vi "semafory.vi"() -> ()   [LabVIEW 2014]
uses:
  semafor.ctl
  #status.ctl
  semafor_tab.ctl
panel:
  in  "stop":bool
  in  "Do":i32
  in  "Od":i32
  out "Semafor S":T1
  out "Semafor  E":T1
  out "Semafor W":T1
  out "Semafor N":T1
  # "Noc"
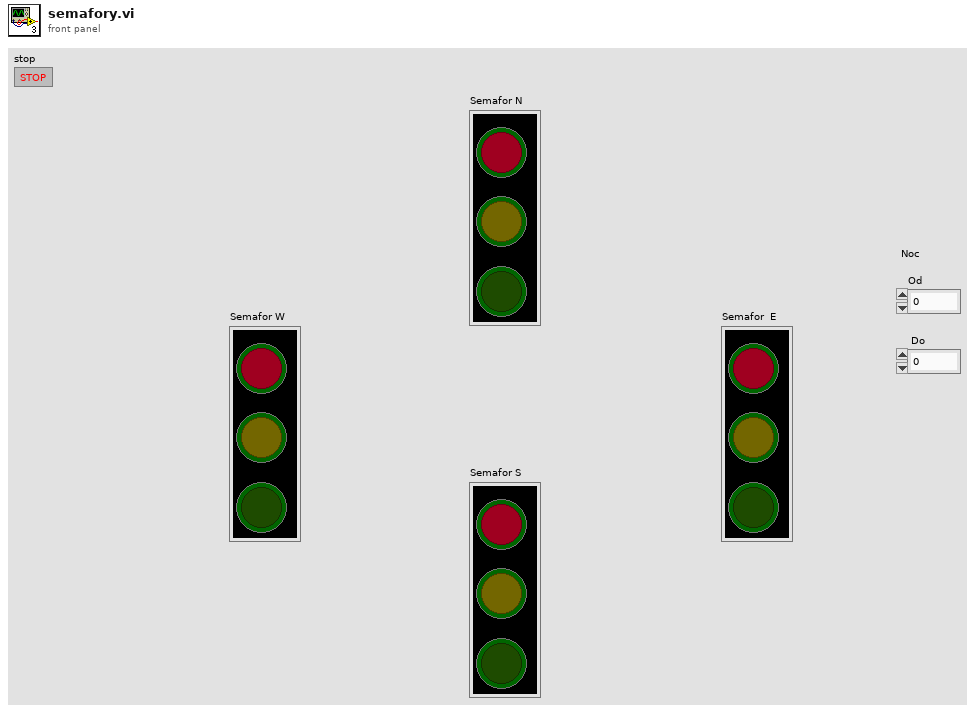
[diagram p1: front panel]
types:
  T1 = typedef "semafor.ctl" = cluster{"Y":bool, "G":bool, "R":bool}
  T2 = typedef "#status.ctl" = enum16{"Error_under_range", "Init", "Idle", "Night", "E-W-R", "E-W-Y", "E-W-G", "N-S-R", "N-S-Y", "N-S-G", "Exit"}
  T3 = typedef "semafor_tab.ctl" = cluster{"N":T1, "S":T1, "W":T1, "E":T1, "Time R ":dbl, "Time  Y":dbl, "Time  G":dbl}
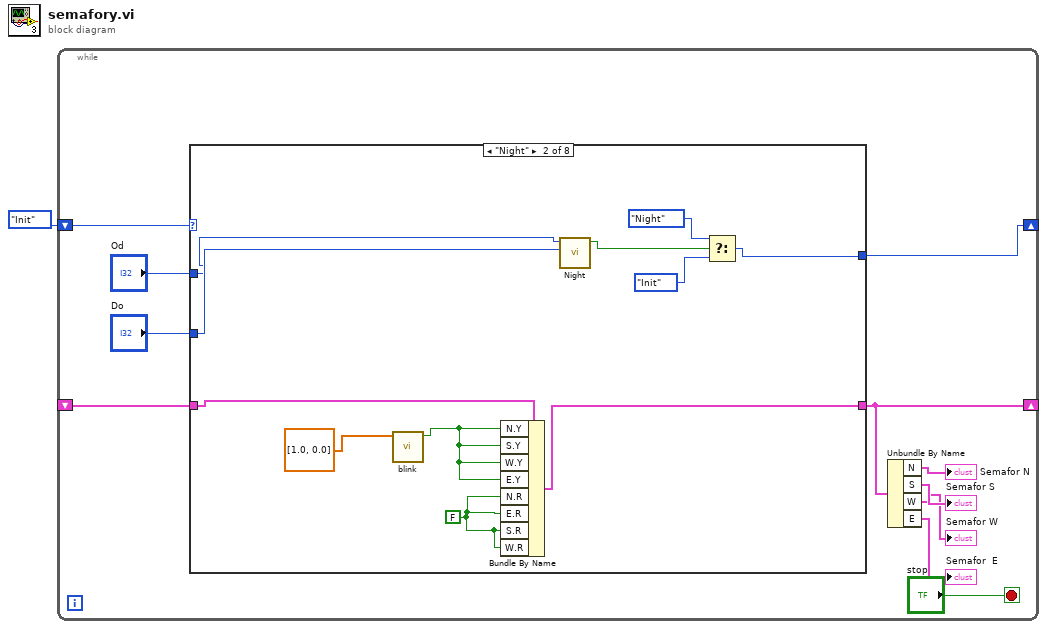
[diagram p0: block diagram]
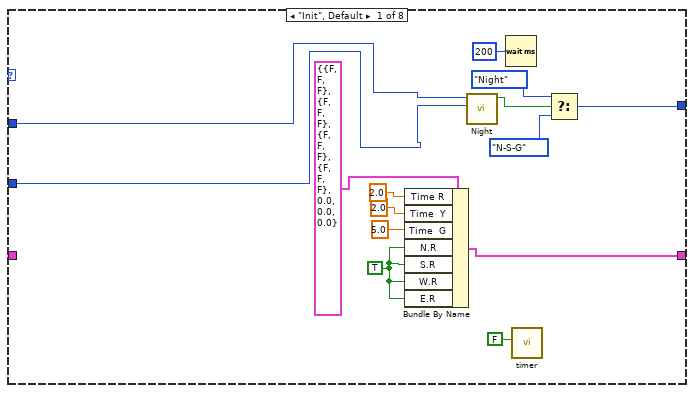
[diagram p2: hidden frame]
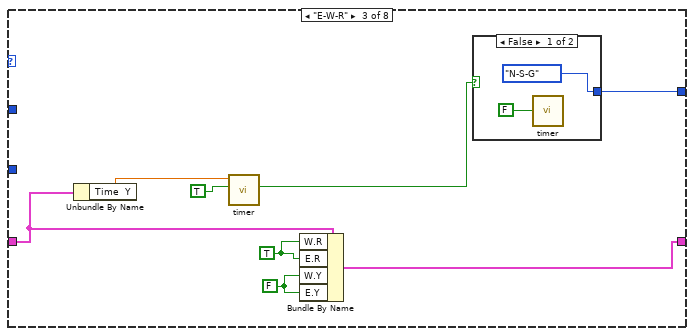
[diagram p3: hidden frame]
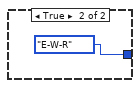
[diagram p4: hidden frame]
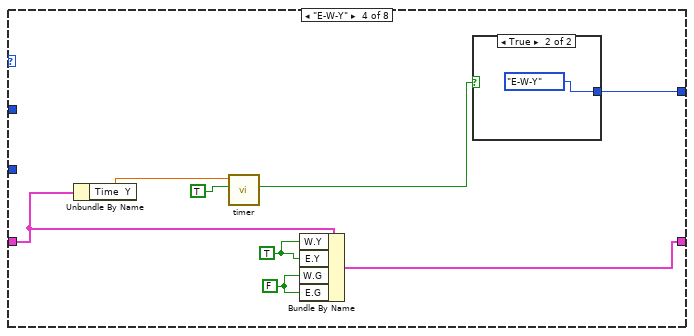
[diagram p5: hidden frame]
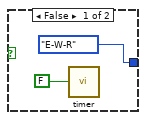
[diagram p6: hidden frame]
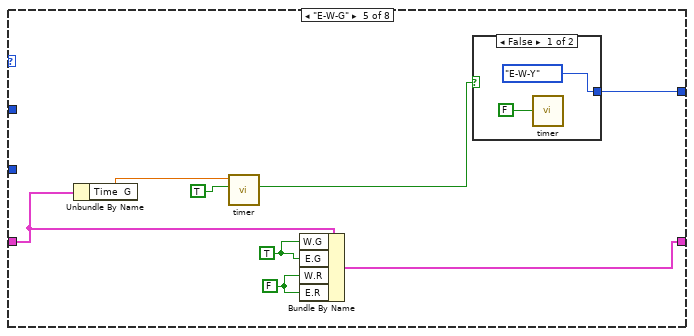
[diagram p7: hidden frame]
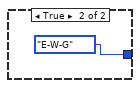
[diagram p8: hidden frame]
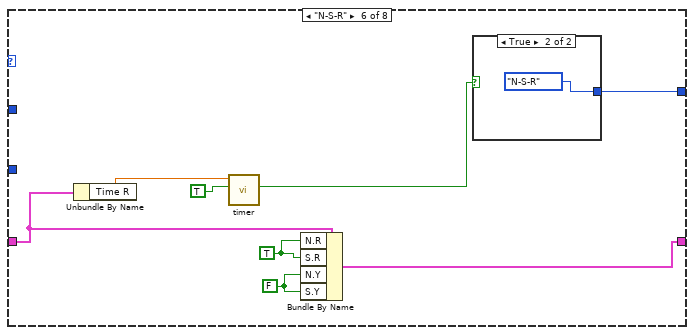
[diagram p9: hidden frame]
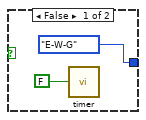
[diagram p10: hidden frame]
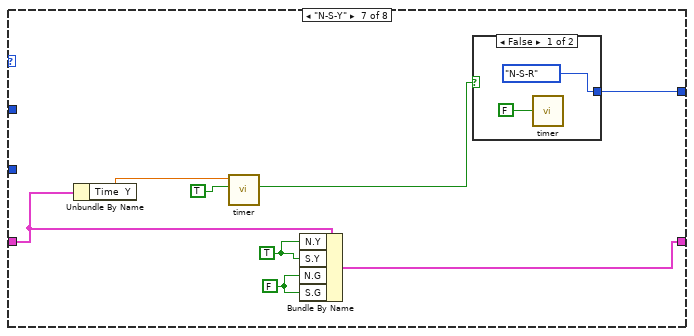
[diagram p11: hidden frame]
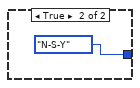
[diagram p12: hidden frame]
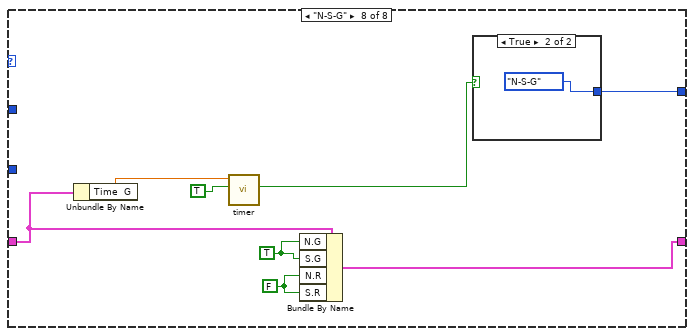
[diagram p13: hidden frame]
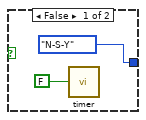
[diagram p14: hidden frame]
diagram:
  n1 = while {
    shift-right: [w11] -> _
    shift-left: #status."Init" ("Enum") -> [w12]
    shift-right: [w10] -> _
    shift-left: _ -> [w5]
    stop <- "stop" stop-if-true
    n2 = case shown="\"Night\"" w12 {
      tunnel: [w17 w27 w39 w50 w61 w72 w83 w94] -> w11
      tunnel: [w16 w33 w38 w49 w60 w71 w82 w93] -> w10
      tunnel: w5 -> [_ w36 w44 w55 w66 w77 w88 w99]
      tunnel: "Do" -> [w14 w30 _ _ _ _ _ _]
      tunnel: "Od" -> [w13 w29 _ _ _ _ _ _]
      frame "Init", Default {
        w22 = TRUE
        n3 = Bundle By Name(cluster=T3 {"N"={"Y"=FALSE, "G"=FALSE, "R"=FALSE}, "S"={"Y"=FALSE, "G"=FALSE, "R"=FALSE}, "W"={"Y"=FALSE, "G"=FALSE, "R"=FALSE}, "E"={"Y"=FALSE, "G"=FALSE, "R"=FALSE}, "Time R "=0.0, "Time  Y"=0.0, "Time  G"=0.0} ("Cluster"), "Time R"=2.0, "Time  Y"=2.0, "Time  G"=5.0, "N.R"=w22, "S.R"=w22, "W.R"=w22, "E.R"=w22) -> (w16:T3)
        n4 = call "Night.vi"("Do"=w14, "Od"=w13) -> ("Noc"=w20:bool)  [unwired: 9 in]
        n5 = Wait (ms)(milliseconds to wait=u32 200) -> ()  [unwired: 1 out]
        n6 = call "timer.vi"("Start/Stop"=FALSE) -> ()  [unwired: 9 in, 2 out]
        n7 = Select(t=#status."Night" ("Enum"), s=w20, f=#status."N-S-G" ("Enum")) -> (s? t:f=w17:T2)
      }
      frame "Night" {
        w34 = FALSE
        n8 = call "blink.vi"("Array"=dbl[] [1.0, 0.0]) -> ("Glitter"=w35:bool)  [unwired: 10 in]
        n9 = Bundle By Name(cluster=w36, "N.Y"=w35, "S.Y"=w35, "W.Y"=w35, "E.Y"=w35, "N.R"=w34, "E.R"=w34, "S.R"=w34, "W.R"=w34) -> (w33:T3)
        n10 = call "Night.vi"("Do"=w30, "Od"=w29) -> ("Noc"=w28:bool)  [unwired: 9 in]
        n11 = Select(t=#status."Night" ("Enum"), s=w28, f=#status."Init" ("Enum")) -> (s? t:f=w27:T2)
      }
      frame "E-W-R" {
        w42 = TRUE
        w43 = FALSE
        n12 = Unbundle By Name(w44) -> ("Time  Y"=w45:dbl)
        n13 = call "timer.vi"("Start/Stop"=TRUE, "Limit"=w45) -> ("Under limit"=w40:bool)  [unwired: 8 in, 1 out]
        n14 = Bundle By Name(cluster=w44, "W.R"=w42, "E.R"=w42, "W.Y"=w43, "E.Y"=w43) -> (w38:T3)
        n15 = case shown="False" w40 {
          tunnel: [#status."N-S-G" ("Enum") #status."E-W-R" ("Enum")] -> w39
          frame False {
            n16 = call "timer.vi"("Start/Stop"=FALSE) -> ()  [unwired: 9 in, 2 out]
          }
          frame True {
          }
        }
      }
      frame "E-W-Y" {
        w53 = TRUE
        w54 = FALSE
        n17 = Unbundle By Name(w55) -> ("Time  Y"=w56:dbl)
        n18 = call "timer.vi"("Start/Stop"=TRUE, "Limit"=w56) -> ("Under limit"=w51:bool)  [unwired: 8 in, 1 out]
        n19 = Bundle By Name(cluster=w55, "W.Y"=w53, "E.Y"=w53, "W.G"=w54, "E.G"=w54) -> (w49:T3)
        n20 = case shown="True" w51 {
          tunnel: [#status."E-W-R" ("Enum") #status."E-W-Y" ("Enum")] -> w50
          frame False {
            n21 = call "timer.vi"("Start/Stop"=FALSE) -> ()  [unwired: 9 in, 2 out]
          }
          frame True {
          }
        }
      }
      frame "E-W-G" {
        w64 = TRUE
        w65 = FALSE
        n22 = Unbundle By Name(w66) -> ("Time  G"=w67:dbl)
        n23 = call "timer.vi"("Start/Stop"=TRUE, "Limit"=w67) -> ("Under limit"=w62:bool)  [unwired: 8 in, 1 out]
        n24 = Bundle By Name(cluster=w66, "W.G"=w64, "E.G"=w64, "W.R"=w65, "E.R"=w65) -> (w60:T3)
        n25 = case shown="False" w62 {
          tunnel: [#status."E-W-Y" ("Enum") #status."E-W-G" ("Enum")] -> w61
          frame False {
            n26 = call "timer.vi"("Start/Stop"=FALSE) -> ()  [unwired: 9 in, 2 out]
          }
          frame True {
          }
        }
      }
      frame "N-S-R" {
        w75 = TRUE
        w76 = FALSE
        n27 = Unbundle By Name(w77) -> ("Time R"=w78:dbl)
        n28 = call "timer.vi"("Start/Stop"=TRUE, "Limit"=w78) -> ("Under limit"=w73:bool)  [unwired: 8 in, 1 out]
        n29 = Bundle By Name(cluster=w77, "N.R"=w75, "S.R"=w75, "N.Y"=w76, "S.Y"=w76) -> (w71:T3)
        n30 = case shown="True" w73 {
          tunnel: [#status."E-W-G" ("Enum") #status."N-S-R" ("Enum")] -> w72
          frame False {
            n31 = call "timer.vi"("Start/Stop"=FALSE) -> ()  [unwired: 9 in, 2 out]
          }
          frame True {
          }
        }
      }
      frame "N-S-Y" {
        w86 = TRUE
        w87 = FALSE
        n32 = Unbundle By Name(w88) -> ("Time  Y"=w89:dbl)
        n33 = call "timer.vi"("Start/Stop"=TRUE, "Limit"=w89) -> ("Under limit"=w84:bool)  [unwired: 8 in, 1 out]
        n34 = Bundle By Name(cluster=w88, "N.Y"=w86, "S.Y"=w86, "N.G"=w87, "S.G"=w87) -> (w82:T3)
        n35 = case shown="False" w84 {
          tunnel: [#status."N-S-R" ("Enum") #status."N-S-Y" ("Enum")] -> w83
          frame False {
            n36 = call "timer.vi"("Start/Stop"=FALSE) -> ()  [unwired: 9 in, 2 out]
          }
          frame True {
          }
        }
      }
      frame "N-S-G" {
        w97 = TRUE
        w98 = FALSE
        n37 = Unbundle By Name(w99) -> ("Time  G"=w100:dbl)
        n38 = call "timer.vi"("Start/Stop"=TRUE, "Limit"=w100) -> ("Under limit"=w95:bool)  [unwired: 8 in, 1 out]
        n39 = Bundle By Name(cluster=w99, "N.G"=w97, "S.G"=w97, "N.R"=w98, "S.R"=w98) -> (w93:T3)
        n40 = case shown="True" w95 {
          tunnel: [#status."N-S-Y" ("Enum") #status."N-S-G" ("Enum")] -> w94
          frame False {
            n41 = call "timer.vi"("Start/Stop"=FALSE) -> ()  [unwired: 9 in, 2 out]
          }
          frame True {
          }
        }
      }
    }
    n42 = Unbundle By Name(w10) -> ("N"=→"Semafor N":T1, "S"=→"Semafor S":T1, "W"=→"Semafor W":T1, "E"=→"Semafor  E":T1)
  }
